vi "Agilent ESG_Configure RF.vi"(8 "error in":errorcluster, 9 "Level":dbl=-90.0 format="%.2f", 10 "Frequency (Hz)":dbl=100000000.0 format="%.2p", 11 "Handle In":variant) -> (0 "error out":errorcluster {"code" format="%.0x"}, 3 "Handle Out":variant)   [LabVIEW 2015]
uses:
  <instrlib>/Agilent ESG Series/Agilent ESG Series.lvlib
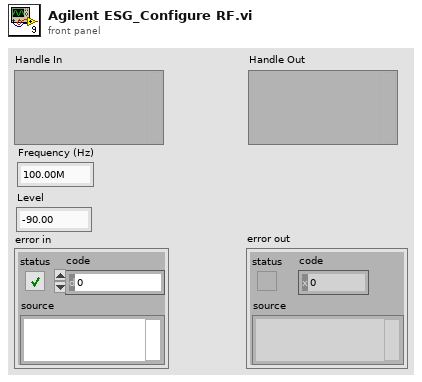
[diagram p1: front panel]
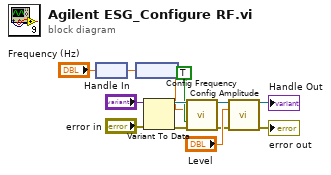
[diagram p0: block diagram]
diagram:
  n1 = node("Frequency (Hz)") -> (w2:dbl[unit])
  n2 = node(w2) -> (w1:dbl)
  n3 = Variant To Data(error in="error in", Variant="Handle In") -> (data=w11:refnum<visa-resource-name>, error out=w10:errorcluster)  [unwired: 1 in]
  n4 = call <instrlib>:"Config Frequency.vi"("VISA Resource Name"=w11, "Frequency (1000.0)"=w1, "Freq Ref (T:ON)"=TRUE ("Enable Reference Frequency (F:Disable)"), "error in (no error)"=w10) -> ("VISA Resource Name Out"=w9:refnum<visa-resource-name>, "error out"=w7:errorcluster)  [unwired: 10 in]
  n5 = call <instrlib>:"Config Amplitude.vi"("VISA Resource Name"=w9, "Amplitude (-135.00)"="Level", "error in (no error)"=w7) -> ("VISA Resource Name Out"=→"Handle Out":refnum<visa-resource-name>, "error out"=→"error out":errorcluster)  [unwired: 11 in]
